vi "SetDefaultParams.vi"(8 "error in (no error)":errorcluster, 11 "NISTSamplerPluginsBase in":refnum<class "SamplerPluginsBase.lvclass">) -> (0 "error out":errorcluster, 3 "NISTSamplerPluginsBase out":refnum<class "SamplerPluginsBase.lvclass">)   [LabVIEW 2014]
uses:
  SamplerPluginsBase.lvclass
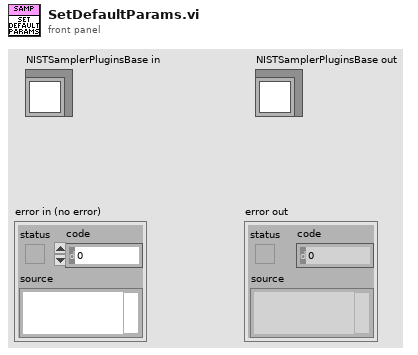
[diagram p1: front panel]
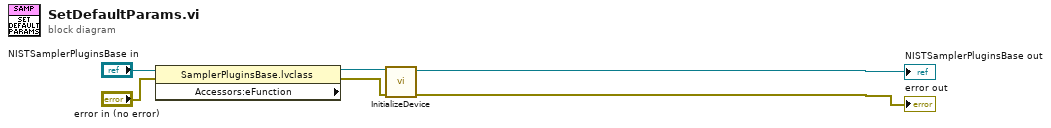
[diagram p0: block diagram]
diagram:
  n1 = property class="SamplerPluginsBase.lvclass" props=["Accessors:eFunction"](reference="NISTSamplerPluginsBase in", error in="error in (no error)") -> (reference out=w2:refnum<class "SamplerPluginsBase.lvclass">, error out=w1:errorcluster)  [unwired: 1 out]
  n2 = call-dynamic "InitializeDevice.vi"("error in (no error)"=w1, "NISTSamplerPluginsBase in"=w2) -> ("error out"=→"error out":errorcluster, "NISTSamplerPluginsBase out"=→"NISTSamplerPluginsBase out":refnum<class "SamplerPluginsBase.lvclass">)  [unwired: 8 in]
